vi "Compare Standard File.vi"(6 "Interactive?":bool, 7 "Baseline Directory":path, 8 "error in":errorcluster, 10 "Results Directory":path, 11 "File Info in":T1) -> (0 "error out":errorcluster, 3 "File Info out":T1)   [LabVIEW 2020, in "Peer Review.lvclass"]
uses:
  Peer Review.lvclass
  TypeDefs/File Info.ctl
  TypeDefs/File State.ctl
  TypeDefs/VI Type.ctl
  Peer Review.lvclass/Peer Review.ctl
  <vilib>/security/Message Digest/API/NI_Message Digest API.lvlib
  <vilib>/security/Message Digest/API/Instances/File/SHA-256 File Checksum.vi
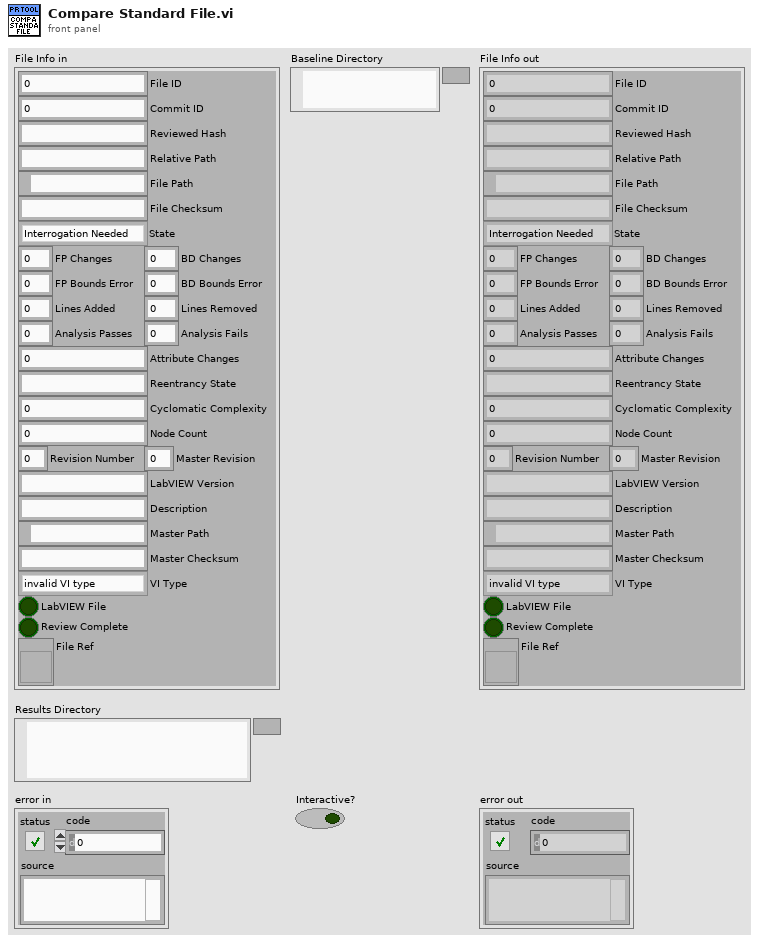
[diagram p1: front panel]
types:
  T1 = typedef "Peer Review.lvclass/File Info.ctl" = cluster{"File ID":i32, "Commit ID":i32, "Reviewed Hash":string, "Relative Path":string, "File Path":path, "File Checksum":string, "State":T2, "FP Changes":i32, "BD Changes":i32, "FP Bounds Error":dbl, "BD Bounds Error":dbl, "Lines Added":i32, "Lines Removed":i32, "Analysis Passes":i32, "Analysis Fails":i32, "Attribute Changes":i32, "Reentrancy State":string, "Cyclomatic Complexity":i32, "Node Count":i32, "Revision Number":u32, "LabVIEW Version":string, "Description":string, "Master Path":path, "Master Checksum":string, "VI Type":T3, "LabVIEW File":bool, "Review Complete":bool, "File Ref":refnum<vi>, "Master Revision":u32}
  T2 = typedef "Peer Review.lvclass/File State.ctl" = enum16{"Interrogation Needed", "Modified", "Deleted", "Added", "Matches Previous", "No Changes", "Moved", "Empty File"}
  T3 = typedef "Peer Review.lvclass/VI Type.ctl" = enum32{"invalid VI type", "Standard VI", "Control VI", "Global VI", "Polymorphic VI", "Configuration VI", "SubSystem", "Facade VI", "Method VI", "Statechart Diagram VI"}
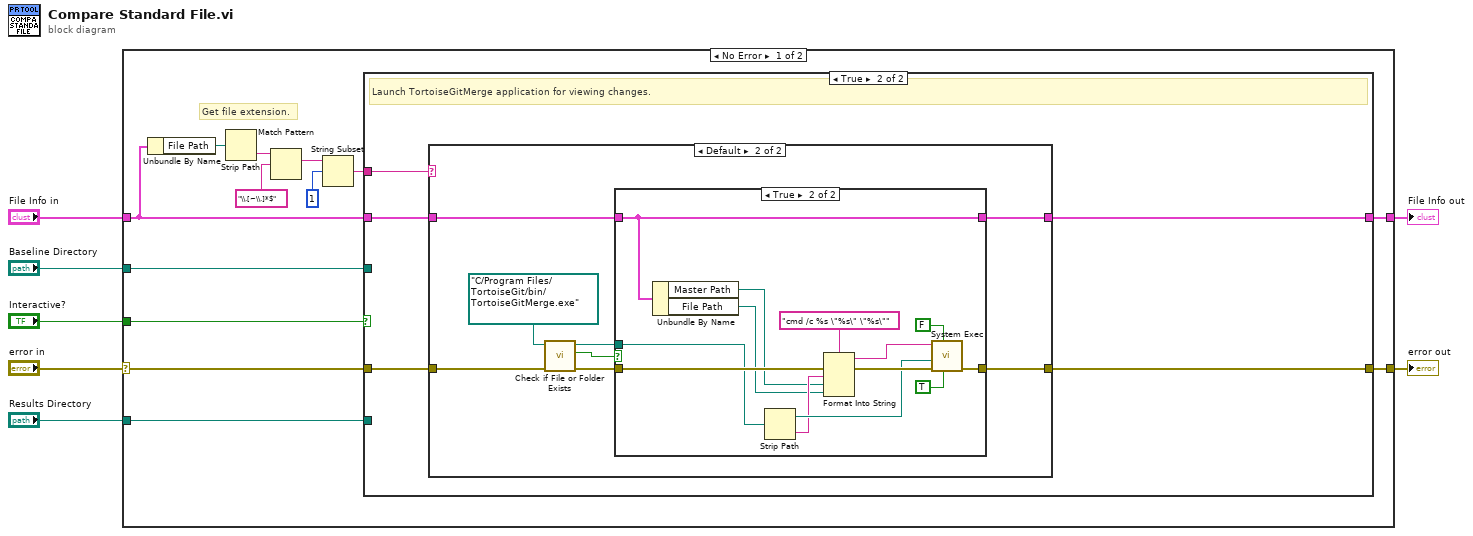
[diagram p0: block diagram]
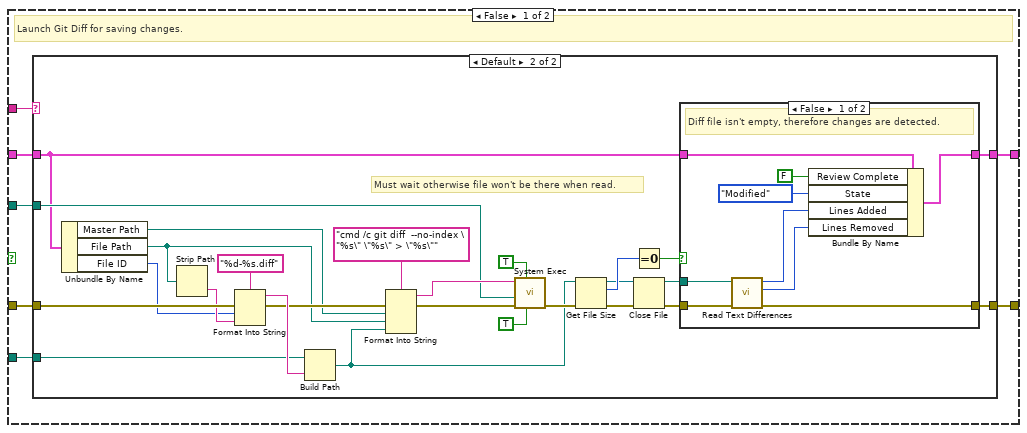
[diagram p2: hidden frame]
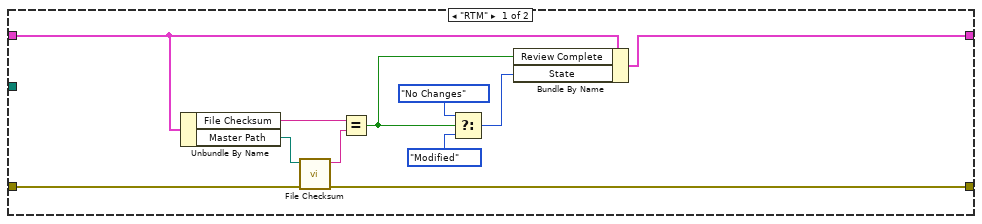
[diagram p3: hidden frame]
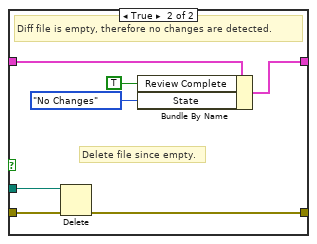
[diagram p4: hidden frame]
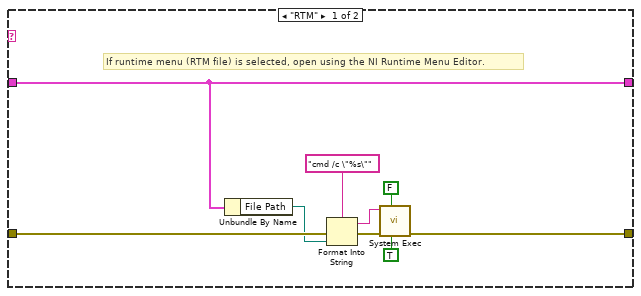
[diagram p5: hidden frame]
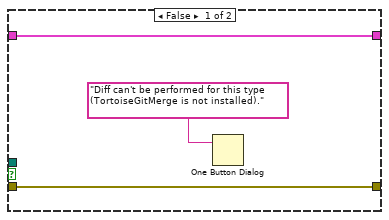
[diagram p6: hidden frame]
diagram:
  n1 = case shown="No Error" "error in" {
    selector: "error in" -> [w20 w119]
    tunnel: [w19 w119] -> w6
    tunnel: [w18 w120] -> w5
    tunnel: "File Info in" -> [w14 w120]
    tunnel: "Interactive?" -> [w17 _]
    tunnel: "Baseline Directory" -> [w16 _]
    tunnel: "Results Directory" -> [w15 _]
    frame No Error {
      # "Get file extension."
      n2 = Unbundle By Name(w14) -> ("File Path"=w9:path)
      n3 = Strip Path(path=w9) -> (name=w12:string)  [unwired: 1 out]
      n4 = Match Pattern(string=w12, regular expression="\\.[~\\.]*$") -> (match substring=w13:string)  [unwired: 4 out]
      n5 = String Subset(string=w13, offset (0)=1) -> (substring=w8:string)  [unwired: 1 out]
      n6 = case shown="True" w17 {
        tunnel: w20 -> [w25 w85]
        tunnel: [w24 w84] -> w19
        tunnel: [w22 w83] -> w18
        tunnel: w14 -> [w23 w82]
        tunnel: w16 -> [w27 _]
        tunnel: w15 -> [w26 _]
        tunnel: w8 -> [w21 w81]
        frame False {
          # "Launch Git Diff for saving changes."
          n7 = case shown="Default" w21 {
            tunnel: w27 -> [_ w59]
            tunnel: w26 -> [_ w56]
            tunnel: w25 -> [w35 w52]
            tunnel: [w36 w48] -> w24
            tunnel: w23 -> [w28 w40]
            tunnel: [w29 w39] -> w22
            frame "RTM" {
              n8 = Unbundle By Name(w28) -> ("File Checksum"=w38:string, "Master Path"=w34:path)
              n9 = call-poly <vilib>:"File Checksum.vi"("error in"=w35, "path"=w34) -> ("error out"=w36:errorcluster, "digest"=w37:string)  [unwired: 8 in]
              n10 = Equal?(x=w38, y=w37) -> (x = y?=w33:bool)
              n11 = Select(t=File_State."No Changes" ("f"), s=w33, f=File_State."Modified") -> (s? t:f=w30:T2)
              n12 = Bundle By Name(cluster=w28, "Review Complete"=w33, "State"=w30) -> (w29:T1)
            }
            frame Default {
              # "Must wait otherwise file won't be there when read."
              n13 = Unbundle By Name(w40) -> ("Master Path"=w54:path, "File Path"=w53:path, "File ID"=w41:i32)
              n14 = Strip Path(path=w53) -> (name=w51:string)  [unwired: 1 out]
              n15 = Format Into String(format string="%d-%s.diff", error in=w52, w41, w51) -> (resulting string=w57:string, error out=w55:errorcluster)  [unwired: 1 in]
              n16 = Build Path(base path=w56, name or relative path=w57) -> (appended path=w47:path)
              n17 = Format Into String(format string="cmd /c git diff  --no-index \"%s\" \"%s\" > \"%s\"", error in=w55, w54, w53, w47) -> (resulting string=w62:string, error out=w64:errorcluster)  [unwired: 1 in]
              n18 = call <vilib>:"System Exec.vi"("run minimized? (F)"=TRUE, "wait until completion? (T)"=TRUE, "error in (no error)"=w64, "working directory"=w59, "command line"=w62) -> ("error out"=w50:errorcluster)  [unwired: 3 in, 3 out]
              n19 = Get File Size(file=w47, error in=w50) -> (refnum out=w46:refnum<file>, size (in bytes)=w49:i64, 0:w45:errorcluster)
              n20 = Equal To 0?(x=w49) -> (x = 0?=w42:bool)
              n21 = Close File(refnum=w46, error in=w45) -> (path=w43:path, error out=w44:errorcluster)
              n22 = case shown="False" w42 {
                tunnel: w44 -> [w71 w80]
                tunnel: [w72 w79] -> w48
                tunnel: w43 -> [w73 w78]
                tunnel: w40 -> [w70 w74]
                tunnel: [w65 w75] -> w39
                frame False {
                  # "Diff file isn't empty, therefore changes are detected."
                  n23 = call "Read Text Differences.vi"("error in"=w71, "Diff File Path"=w73) -> ("error out"=w72:errorcluster, "Removed"=w66:i32, "Added"=w67:i32)  [unwired: 7 in]
                  n24 = Bundle By Name(cluster=w70, "Review Complete"=FALSE ("Review Complete?"), "State"=File_State."Modified" ("f"), "Lines Added"=w67, "Lines Removed"=w66) -> (w65:T1)
                }
                frame True {
                  # "Delete file since empty."
                  # "Diff file is empty, therefore no changes are detected."
                  n25 = Delete(path (use dialog)=w78, error in=w80) -> (error out=w79:errorcluster)  [unwired: 3 in, 2 out]
                  n26 = Bundle By Name(cluster=w74, "Review Complete"=TRUE ("Review Complete?"), "State"=File_State."No Changes") -> (w75:T1)
                }
              }
            }
          }
        }
        frame True {
          # "Launch TortoiseGitMerge application for viewing changes."
          n27 = case shown="Default" w81 {
            tunnel: w85 -> [w89 w102]
            tunnel: [w88 w101] -> w84
            tunnel: [w87 w100] -> w83
            tunnel: w82 -> [w87 w99]
            frame "RTM" {
              # "If runtime menu (RTM file) is selected, open using the NI Runtime Menu Editor."
              n28 = Unbundle By Name(w87) -> ("File Path"=w86:path)
              n29 = Format Into String(format string="cmd /c \"%s\"", error in=w89, w86) -> (resulting string=w92:string, error out=w91:errorcluster)  [unwired: 1 in]
              n30 = call <vilib>:"System Exec.vi"("run minimized? (F)"=TRUE, "wait until completion? (T)"=FALSE, "error in (no error)"=w91, "command line"=w92) -> ("error out"=w88:errorcluster)  [unwired: 4 in, 3 out]
            }
            frame Default {
              n31 = call <vilib>:"Check if File or Folder Exists.vi"("error in (no error)"=w102, "path"=path "C:/Program Files/TortoiseGit/bin/TortoiseGitMerge.exe" ("working directory")) -> ("error out"=w98:errorcluster, "file or folder exists?"=w96:bool, "dup path"=w95:path)  [unwired: 7 in]
              n32 = case shown="True" w96 {
                tunnel: w98 -> [w105 w117]
                tunnel: [w105 w112] -> w101
                tunnel: [w104 w106] -> w100
                tunnel: w99 -> [w104 w106]
                tunnel: w95 -> [_ w116]
                frame False {
                  n33 = One Button Dialog(message="Diff can't be performed for this type (TortoiseGitMerge is not installed).") -> ()  [unwired: 1 in, 1 out]
                }
                frame True {
                  n34 = Unbundle By Name(w106) -> ("Master Path"=w110:path, "File Path"=w109:path)
                  n35 = Strip Path(path=w116) -> (stripped path=w114:path, name=w111:string)
                  n36 = Format Into String(format string="cmd /c %s \"%s\" \"%s\"", error in=w117, w111, w110, w109) -> (resulting string=w113:string, error out=w118:errorcluster)  [unwired: 1 in]
                  n37 = call <vilib>:"System Exec.vi"("run minimized? (F)"=TRUE, "wait until completion? (T)"=FALSE, "error in (no error)"=w118, "working directory"=w114, "command line"=w113) -> ("error out"=w112:errorcluster)  [unwired: 3 in, 3 out]
                }
              }
            }
          }
        }
      }
    }
    frame Error {
    }
  }
  "File Info out" <- w5
  "error out" <- w6
